vi "ArrayLast_S.vi"(11 "1D Array In":string[](array[string])) -> (0 "Last":string, 1 "Head of Array":string[](array[string]))   [LabVIEW 2013]
doc: "Splits an array into the head and the last element. Throws error if input array is empty."
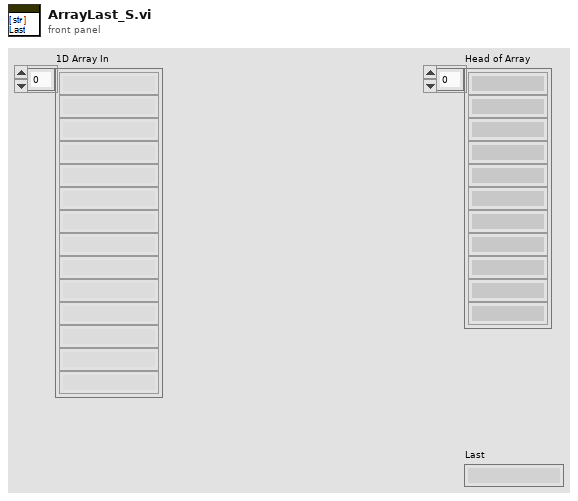
[diagram p1: front panel]
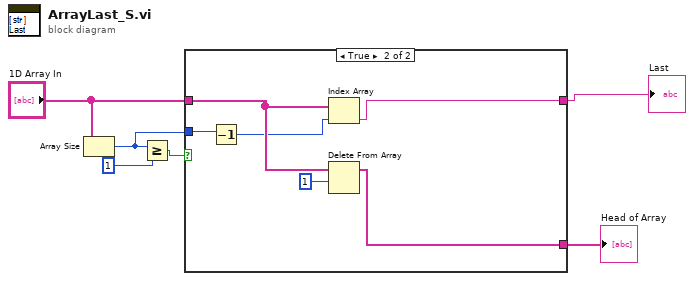
[diagram p0: block diagram]
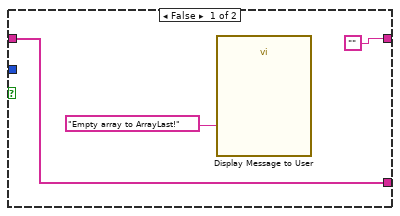
[diagram p2: hidden frame]
diagram:
  n1 = Array Size(array="1D Array In") -> (size(s)=w2:i32)
  n2 = Greater Or Equal?(x=w2, y=1) -> (x >= y?=w5:bool)
  n3 = case shown="True" w5 {
    tunnel: "1D Array In" -> [w9 w14]
    tunnel: ["" w10] -> w1
    tunnel: [w9 w13] -> w3
    tunnel: w2 -> [_ w12]
    frame False {
      n4 = call "Display Message to User"("Message"="Empty array to ArrayLast!") -> ()  [unwired: 9 in, 2 out]
    }
    frame True {
      n5 = Decrement(x=w12) -> (x-1=w11:i32)
      n6 = Index Array(array=w14, index=w11) -> (element=w10:string)
      n7 = Delete From Array(array=w14, length=1) -> (array with subset deleted=w13:string[])  [unwired: 1 in, 1 out]
    }
  }
  "Head of Array" <- w3
  "Last" <- w1
